vi "BME280_Temp_Druck_Feuchtigkeit VI.vi"(8 "error in (no error)":errorcluster, 11 "Stop Button":bool) -> (0 "error out":errorcluster, 1 "Druck (bar)":dbl format="%.7f", 2 "Luftfeuchtigkeit %rH":dbl format="%.7f", 3 "Temp (°C)":dbl format="%.7f")   [LabVIEW 2018]
doc: "The myRIO Project template acquires acceleration data from the onboard accelerometer and displays the changes of acceleration values in a waveform chart."
uses:
  <vilib>/myRIO/Instrument Drivers/Onboard IO/I2C/typedefs/I2C User Configuration.ctl
  <vilib>/myRIO/Instrument Drivers/Onboard IO/I2C/typedefs/I2C Transfer Rate.ctl
  <vilib>/myRIO/Instrument Drivers/Onboard IO/I2C/typedefs/I2C Reference.ctl
  <vilib>/myRIO/Common/Instrument Driver Framework/Utilities/typedefs/myRIO Generic Hardware Reference.ctl
  <vilib>/myRIO/Common/Instrument Driver Framework/Utilities/typedefs/Hardware Version Enum.ctl
  <vilib>/myRIO/Common/Instrument Driver Framework/Utilities/typedefs/myRIO v1.0 Reference.ctl
  <vilib>/myRIO/Common/Instrument Driver Framework/Utilities/typedefs/Generic FPGA Reference.ctl
  <vilib>/myRIO/Common/Instrument Driver Framework/myRIO v1.0/I2C/typedefs/I2C Channels Enum.ctl
  <vilib>/myRIO/Instrument Drivers/Onboard IO/I2C/typedefs/I2C Configuration.ctl
  <vilib>/userdefined/High Color/nirio_resource_hc.ctl
  <vilib>/myRIO/Common/Instrument Driver Framework/myRIO v1.0/I2C/vis/myRIO v1.1 Open I2C.vi
  <vilib>/myRIO/Common/Instrument Driver Framework/Utilities/vis/Validate Channels.vi
  <vilib>/myRIO/Common/Instrument Driver Framework/myRIO v1.0/I2C/vis/myRIO v1.0 Reserve I2C.vi
  <vilib>/myRIO/Common/Instrument Driver Framework/myRIO v1.0/I2C/vis/myRIO v1.0 Close I2C.vi
  <vilib>/myRIO/Common/Instrument Driver Framework/myRIO v1.0/I2C/vis/myRIO v1.0 Build MUX Configuration I2C.vi
  <vilib>/myRIO/Common/Instrument Driver Framework/myRIO v1.0/Resource Manager/vis/myRIO v1.0 Reserve Channel List.vi
  <vilib>/myRIO/Common/Instrument Driver Framework/myRIO v1.0/I2C/vis/myRIO v1.0 Unreserve I2C.vi
  <vilib>/myRIO/Common/Instrument Driver Framework/myRIO v1.0/Resource Manager/vis/myRIO v1.0 Create Configuration List.vi
  <vilib>/myRIO/Common/Instrument Driver Framework/myRIO v1.0/Resource Manager/vis/myRIO v1.0 Reserve Channel.vi
  <vilib>/myRIO/Common/Instrument Driver Framework/myRIO v1.0/Resource Manager/vis/myRIO v1.0 Unreserve Channel.vi
  <vilib>/myRIO/Common/Instrument Driver Framework/myRIO v1.0/Resource Manager/vis/myRIO v1.0 Unreserve Channel List.vi
  <vilib>/myRIO/Common/Instrument Driver Framework/myRIO v1.0/Resource Manager/vis/myRIO v1.0 Build Mutex Name.vi
  <vilib>/Utility/VariantDataType/GetNumericInfo.vi
  <vilib>/Utility/error.llb/Error Cluster From Error Code.vi
  <vilib>/myRIO/Common/Instrument Driver Framework/myRIO v1.0/myRIO v1.1 Open.vi
  <vilib>/myRIO/Common/Instrument Driver Framework/Utilities/vis/IO Manager.vi
  <vilib>/myRIO/Common/Instrument Driver Framework/Utilities/vis/Configuration Manager.vi
  <vilib>/myRIO/Common/Instrument Driver Framework/myRIO v1.0/Resource Manager/vis/myRIO v1.0 Configure IO.vi
  <vilib>/myRIO/Common/Instrument Driver Framework/myRIO v1.0/myRIO v1.0 Close.vi
  <vilib>/myRIO/Common/Instrument Driver Framework/myRIO v1.0/I2C/vis/myRIO v1.0 Configure I2C.vi
  <vilib>/myRIO/Common/Instrument Driver Framework/myRIO v1.0/I2C/vis/myRIO v1.0 Shutdown I2C.vi
  <vilib>/myRIO/Instrument Drivers/Onboard IO/I2C/vis/myRIO I2C Open.xnode
  <vilib>/myRIO/Instrument Drivers/Onboard IO/I2C/I2C.lvlib
panel:
  out "ADC RAW PRESSURE":u32 format="%020b"
  out "Bytes Read Pressure":u8[](array[numeric]) format="%08b"
  out "Bytes Read Humidity":u8[](array[numeric]) format="%08b"
  out "ADC RAW HUMIDITY":u32 format="%016b"
  out "ADC RAW TEMP":i32 format="%020b"
  out "Bytes Read Temp":u8[](array[numeric]) format="%08b"
  out "ChipID":u8[](array[numeric]) format="%x"
  # "BME280"
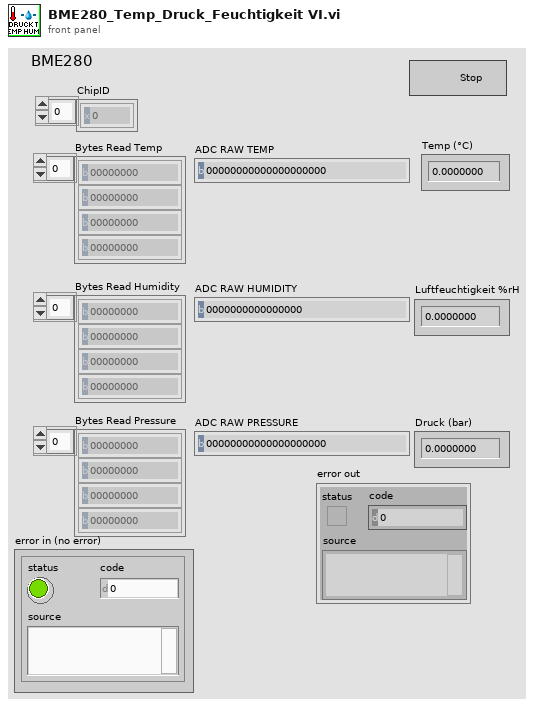
[diagram p1: front panel]
types:
  T1 = typedef "I2C.lvlib/I2C User Configuration.ctl" = cluster{"I2C Transfer Rate":T2}
  T2 = typedef "I2C.lvlib/I2C Transfer Rate.ctl" = enum16{"Standard mode (100 kbps)", "Fast mode (400 kbps)"}
  T3 = typedef "nirio_resource_hc.ctl" = tag
  T4 = typedef "Hardware Version Enum.ctl" = enum16{"Unknown", "myRIO-1900", "myRIO-1950", "roboRIO", "NI ELVIS RIO CM", "ELVIS III"}
  T5 = typedef "I2C.lvlib/I2C Reference.ctl" = cluster{"myRIO Reference":T6, "I2C Channels Enum":T9, "I2C Configuration":T10}
  T6 = typedef "myRIO Generic Hardware Reference.ctl" = cluster{"myRIO Model":T4, "myRIO Hardware Reference":T7}
  T7 = typedef "myRIO v1.0 Reference.ctl" = cluster{"Generic FPGA Reference":T8, "Allow multiple opens":bool}
  T8 = typedef "Generic FPGA Reference.ctl" = refnum<k20>
  T9 = typedef "I2C Channels Enum.ctl" = enum16{"Not Connected", "A/I2C", "B/I2C", "I2C/I2C"}
  T10 = typedef "I2C.lvlib/I2C Configuration.ctl" = cluster{"I2C Transfer Rate":T2}
  T11 = typedef "calib_data.ctl" = cluster{"dig_T1":u16, "dig_T2":i16, "dig_T3":i16, "dig_P1":u16, "dig_P2":i16, "dig_P3":i16, "dig_P4":i16, "dig_P5":i16, "dig_P6":i16, "dig_P7":i16, "dig_P8":i16, "dig_P9":i16, "dig_H1":u8, "dig_H2":i16, "dig_H3":u8, "dig_H4":i16, "dig_H5":i16, "dig_H6":i8}
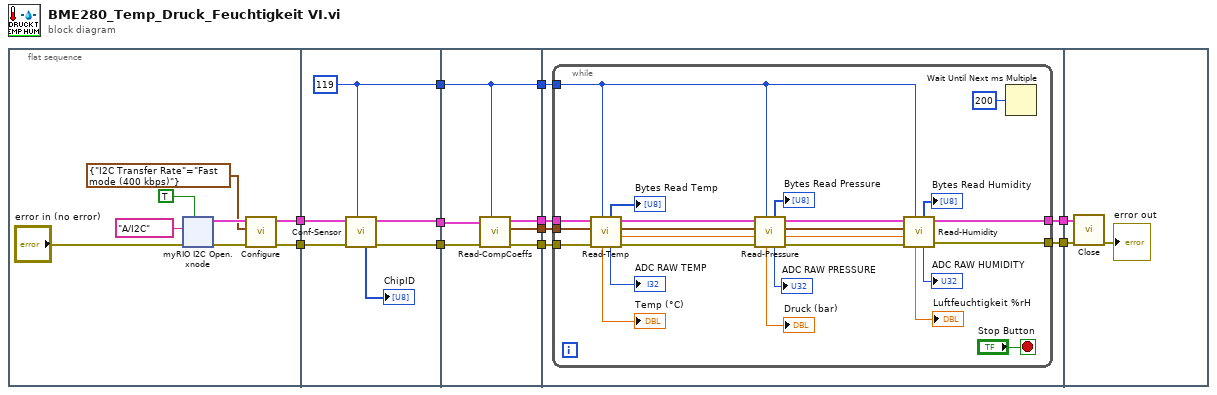
[diagram p0: block diagram]
diagram:
  n1 = flat-sequence {
    tunnel: [w15] -> w11
    tunnel: [w14] -> w10
    tunnel: w11 -> [w38]
    tunnel: w10 -> [w40]
    tunnel: [w41] -> w9
    tunnel: [w39] -> w8
    tunnel: [w37] -> w3
    tunnel: w9 -> [w47]
    tunnel: w8 -> [w44]
    tunnel: [w44] -> w7
    tunnel: [w46] -> w6
    tunnel: [w45] -> w5
    tunnel: [w43] -> w4
    tunnel: w3 -> [w42]
    tunnel: w7 -> [w53]
    tunnel: w6 -> [w52]
    tunnel: w5 -> [w51]
    tunnel: w4 -> [w50]
    tunnel: [w49] -> w2
    tunnel: [w48] -> w1
    tunnel: w2 -> [w81]
    tunnel: w1 -> [w80]
    frame #0 {
      n2 = xnode "myRIO I2C Open.xnode"("error in (no error)"="error in (no error)", "Allow multiple opens?"=TRUE, "Channel Name"=tag "A/I2C") -> ("error out"=w18:errorcluster, "I2C Ref Out"=w19:T5)
      n3 = call <vilib>:"Configure.vi"("error in (no error)"=w18, "I2C User Configuration"=T1 {"I2C Transfer Rate"=enum."Fast mode (400 kbps)"}, "I2C Ref In"=w19) -> ("error out"=w14:errorcluster, "I2C Ref Out"=w15:T5)  [unwired: 7 in]
    }
    frame #1 {
      w39 = u8 119 ("Slave Address (7-bit)")
      n4 = call "Conf-Sensor.vi"("Slave Address (7-bit)"=w39, "error in (no error)"=w40, "I2C Ref Out in"=w38) -> ("error out"=w41:errorcluster, "I2C Ref Out out"=w37:T5, "ChipID"=→"ChipID":u8[])  [unwired: 6 in]
    }
    frame #2 {
      n5 = call "Read-CompCoeffs.vi"("Slave Address (7-bit)"=w44, "error in (no error)"=w47, "I2C Ref Out in"=w42) -> ("error out"=w45:errorcluster, "Comp Coeffs Out"=w43:T11, "I2C Ref Out out"=w46:T5)  [unwired: 6 in]
    }
    frame #3 {
      n6 = while {
        tunnel: w53 -> [w60]
        tunnel: w52 -> [w76]
        tunnel: w51 -> [w75]
        tunnel: w50 -> [w74]
        tunnel: [w56] -> w49
        tunnel: [w55] -> w48
        stop <- "Stop Button" stop-if-true
        n7 = call "Read-Temp.vi"("Slave Address (7-bit)"=w60, "error in (no error)"=w75, "Comp Coeffs"=w74, "I2C Ref Out in"=w76) -> ("error out"=w68:errorcluster, "T_fine"=w69:dbl, "Comp Coeffs Out"=w70:T11, "I2C Ref Out out"=w71:T5, "ADC RAW TEMP"=→"ADC RAW TEMP":i32, "Bytes Read Temp"=→"Bytes Read Temp":u8[], "T"=→"Temp (°C)":dbl)  [unwired: 1 in]
        n8 = call "Read-Pressure.vi"("Slave Address (7-bit)"=w60, "error in (no error)"=w68, "T_fine"=w69, "Comp Coeffs"=w70, "I2C Ref Out in"=w71) -> ("error out"=w64:errorcluster, "T_fine Out"=w61:dbl, "Comp Coeffs Out"=w62:T11, "I2C Ref Out"=w63:T5, "ADC RAW PRESSURE"=→"ADC RAW PRESSURE":u32, "Bytes Read"=→"Bytes Read Pressure":u8[], "p"=→"Druck (bar)":dbl)
        n9 = call "Read-Humidity.vi"("Slave Address (7-bit)"=w60, "error in (no error)"=w64, "T_fine"=w61, "Comp Coeffs"=w62, "I2C Ref In"=w63) -> ("error out"=w55:errorcluster, "I2C Ref Out"=w56:T5, "ADC RAW HUMIDITY"=→"ADC RAW HUMIDITY":u32, "Bytes Read"=→"Bytes Read Humidity":u8[], "Humidity"=→"Luftfeuchtigkeit %rH":dbl)  [unwired: 2 in]
        n10 = Wait Until Next ms Multiple(millisecond multiple=u32 200) -> ()  [unwired: 1 out]
      }
    }
    frame #4 {
      n11 = call <vilib>:"Close.vi"("error in (no error)"=w80, "I2C Ref In"=w81) -> ("error out"=→"error out":errorcluster)  [unwired: 9 in]
    }
  }
